vi "AI AND AO Clock Sync.vi"(7 "AI In":refnum<k21>[](array[refnum]), 8 "error in (no error)":errorcluster, 9 "RefClk.Src":tag, 10 "USB-4431?":bool, 11 "AO in":refnum<k21>[](array[refnum])) -> (0 "error out":errorcluster, 1 "SampClk.Timebase.Rate":dbl, 2 "AO Out":refnum<k21>[](array[refnum]), 3 "AI Out":refnum<k21>[](array[refnum]), 5 "SampQuant.SampPerChan":dbl)   [LabVIEW 2016]
uses:
  <vilib>/DAQmx/configure/trigger.llb/DAQmx Start Trigger (Digital Edge).vi
  <resource>/objmgr/daqmx.rc
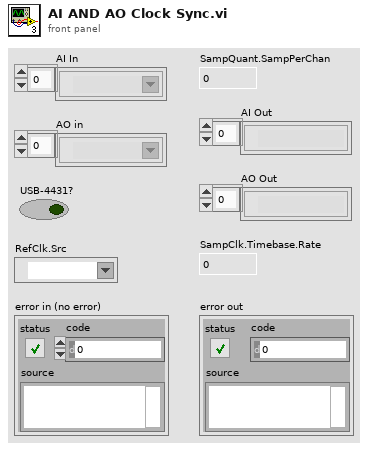
[diagram p1: front panel]
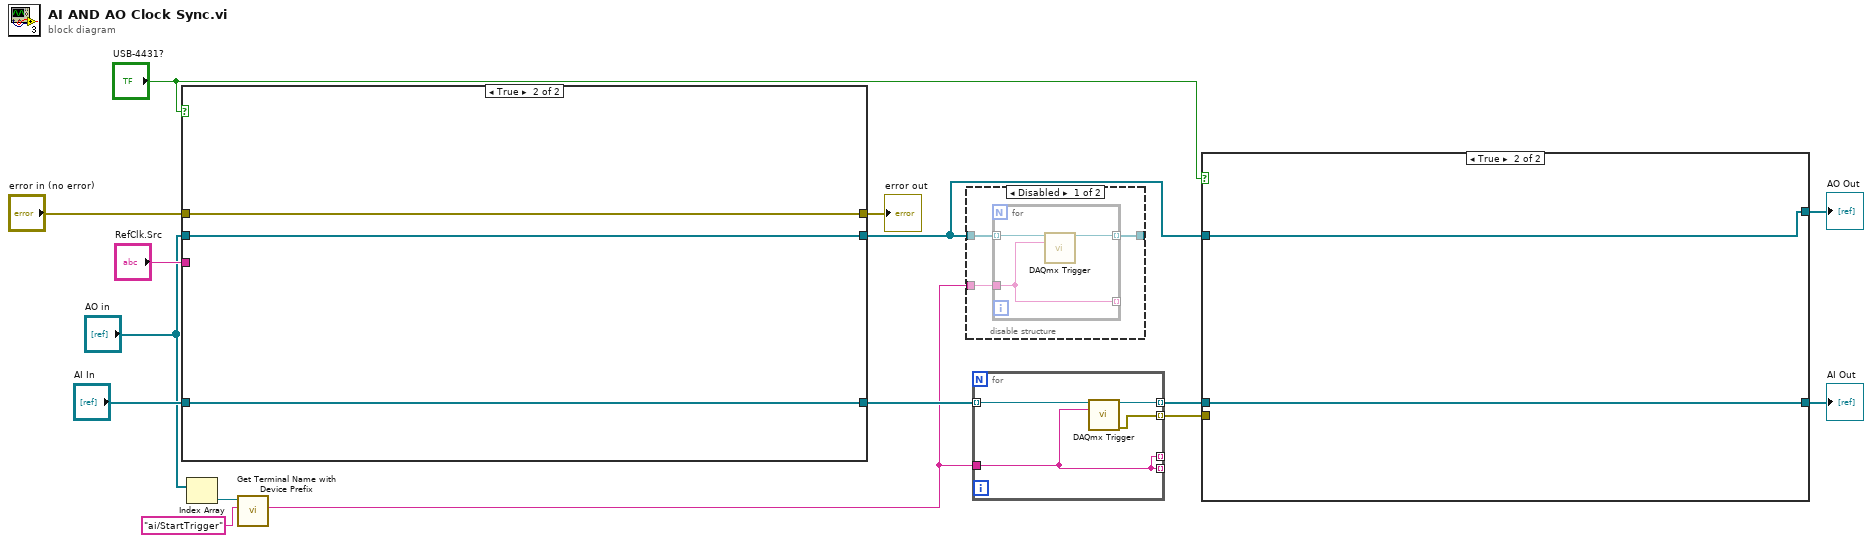
[diagram p0: block diagram]
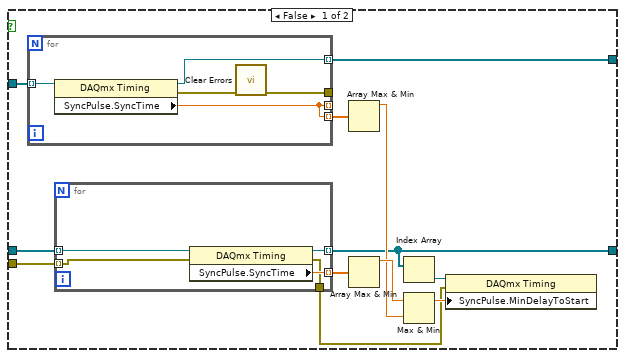
[diagram p3: hidden frame]
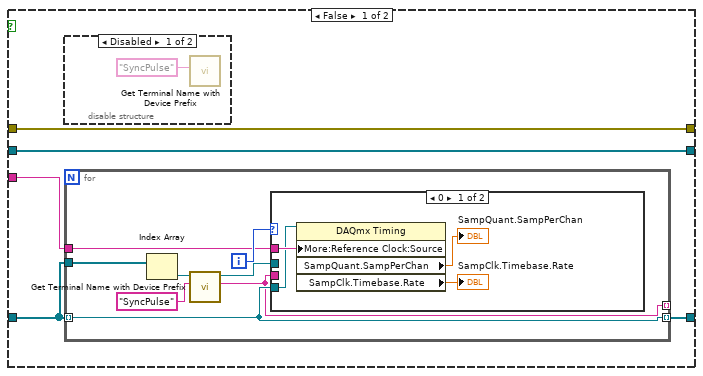
[diagram p4: hidden frame]
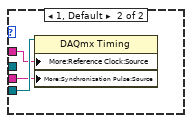
[diagram p6: hidden frame]
diagram:
  n1 = case shown="True" "USB-4431?" {
    tunnel: "RefClk.Src" -> [w19 _]
    tunnel: "AI In" -> [w20 w39]
    tunnel: [w16 w39] -> w6
    tunnel: "AO in" -> [w18 w38]
    tunnel: [w17 w37] -> w14
    tunnel: [w18 w38] -> w2
    tunnel: "error in (no error)" -> [w17 w37]
    frame False {
      n2 = disable-structure shown="Disabled" {
        frame Disabled {
          n3 = call "Get Terminal Name with Device Prefix.vi"("Local Terminal Name"="SyncPulse") -> ()  [unwired: 8 in, 3 out]
        }
        frame Enabled {
        }
      }
      n4 = for {
        tunnel: w20 -> [w26] mode=indexing
        tunnel: w19 -> [w27]
        tunnel: [w26] -> w16 mode=indexing
        tunnel: w20 -> [w25]
        tunnel: [w22] -> _ mode=indexing
        i -> [w29]
        n5 = Index Array(array=w25) -> (element=w24:refnum<k21>)  [unwired: 1 in]
        n6 = call "Get Terminal Name with Device Prefix.vi"("Local Terminal Name"="SyncPulse", "task/channels in"=w24) -> ("Terminal Name with Device Prefix"=w22:tag, "task out"=w23:refnum<k21>)  [unwired: 7 in, 1 out]
        n7 = case shown="0" w29 {
          tunnel: w26 -> [w32 w36]
          tunnel: w22 -> [_ w35]
          tunnel: w27 -> [w33 w34]
          tunnel: w23 -> [_ _]
          frame 0 {
            n8 = property class="DAQmx Timing"(reference=w32, "More:Reference Clock:Source"=w33) -> ("SampQuant.SampPerChan"=→"SampQuant.SampPerChan":dbl, "SampClk.Timebase.Rate"=→"SampClk.Timebase.Rate":dbl)  [unwired: 1 in, 2 out]
          }
          frame 1, Default {
            n9 = property class="DAQmx Timing"(reference=w36, "More:Reference Clock:Source"=w34, "More:Synchronization Pulse:Source"=w35) -> ()  [unwired: 1 in, 2 out]
          }
        }
      }
    }
    frame True {
    }
  }
  "error out" <- w14
  n10 = Index Array(array="AO in") -> (element=w9:refnum<k21>)  [unwired: 1 in]
  n11 = call "Get Terminal Name with Device Prefix.vi"("Local Terminal Name"="ai/StartTrigger", "task/channels in"=w9) -> ("Terminal Name with Device Prefix"=w4:tag)  [unwired: 7 in, 2 out]
  n12 = disable-structure shown="Disabled" {
    disable-tunnel: w4 -> [w42 _]
    disable-tunnel: w2 -> [w41 _]
    disable-tunnel: [w40 _] -> _
    frame Disabled {
      n13 = for {
        tunnel: w41 -> [w45] mode=indexing
        tunnel: [w44] -> w40 mode=indexing
        tunnel: [w43] -> _ mode=indexing
        tunnel: w42 -> [w43]
        n14 = call-poly <vilib>:"DAQmx Trigger.vi"("task/channels in"=w45, "source"=w43) -> ("task out"=w44:refnum<k21>)  [unwired: 12 in, 1 out]
      }
    }
    frame Enabled {
    }
  }
  n15 = for {
    tunnel: w6 -> [w49] mode=indexing
    tunnel: [w48] -> w5 mode=indexing
    tunnel: [w47] -> _ mode=indexing
    tunnel: [w47] -> _ mode=indexing
    tunnel: w4 -> [w47]
    tunnel: [w46] -> w1 mode=indexing
    n16 = call-poly <vilib>:"DAQmx Trigger.vi"("task/channels in"=w49, "source"=w47) -> ("task out"=w48:refnum<k21>, "error out"=w46:errorcluster)  [unwired: 12 in]
  }
  n17 = case shown="True" "USB-4431?" {
    tunnel: w5 -> [w55 w73]
    tunnel: [w53 w73] -> w8
    tunnel: [w52 w72] -> w7
    tunnel: w2 -> [w54 w72]
    tunnel: w1 -> [w51 _]
    frame False {
      n18 = for {
        tunnel: w54 -> [w66] mode=indexing
        tunnel: [w65] -> w52 mode=indexing
        tunnel: [w62] -> _ mode=indexing
        tunnel: [w63] -> _
        tunnel: [w62] -> w57 mode=indexing
        n19 = property class="DAQmx Timing"(reference=w66) -> (reference out=w65:refnum<k21>, error out=w64:errorcluster, "SyncPulse.SyncTime"=w62:dbl)  [unwired: 1 in]
        n20 = call <vilib>:"Clear Errors.vi"("error in (no error)"=w64) -> ("error out"=w63:errorcluster)  [unwired: 5 in, 1 out]
      }
      n21 = for {
        tunnel: w55 -> [w71] mode=indexing
        tunnel: [w70] -> w61 mode=indexing
        tunnel: [w69] -> w53 mode=indexing
        tunnel: w51 -> [w68] mode=indexing
        tunnel: [w67] -> w50
        n22 = property class="DAQmx Timing"(reference=w71, error in=w68) -> (reference out=w69:refnum<k21>, error out=w67:errorcluster, "SyncPulse.SyncTime"=w70:dbl)
      }
      n23 = Array Max & Min(array=w57) -> (max value=w56:dbl)  [unwired: 3 out]
      n24 = Array Max & Min(array=w61) -> (max value=w59:dbl)  [unwired: 3 out]
      n25 = Index Array(array=w53) -> (element=w60:refnum<k21>)  [unwired: 1 in]
      n26 = Max & Min(x=w59, y=w56) -> (max(x,y)=w58:dbl)  [unwired: 1 out]
      n27 = property class="DAQmx Timing"(reference=w60, error in=w50, "SyncPulse.MinDelayToStart"=w58) -> ()  [unwired: 2 out]
    }
    frame True {
    }
  }
  "AO Out" <- w7
  "AI Out" <- w8
